vi "Word_Append_Or_Create_Table.vi"(7 "MS Office parameters":T1, 8 "error in (no error)":errorcluster, 9 "Data":string[][](array[string]), 10 "Column Headers":string[](array[string]), 11 "Report in":refnum<class "NI_report.lvclass">) -> (0 "error out":errorcluster, 3 "report out":refnum<class "NI_report.lvclass">)   [LabVIEW 2017, in "NI_ReportGenerationToolkit.lvlib"]
uses:
  <vilib>/addons/_office/NI_ReportGenerationToolkit.lvlib
  <vilib>/Utility/NIReport.llb/NI_report.lvclass
  <vilib>/Utility/NIReport.llb/Word/NI_Word.lvclass
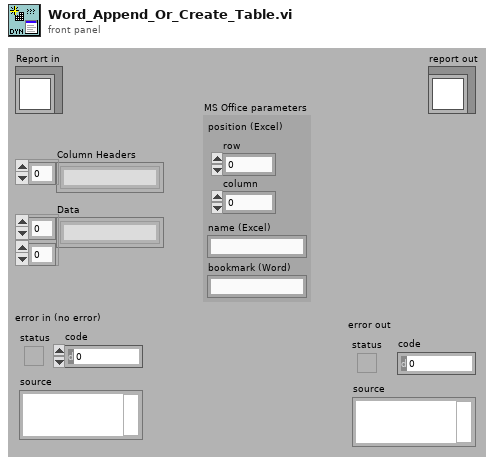
[diagram p1: front panel]
types:
  T1 = cluster{"position (Excel)":cluster{"row":i32, "column":i32}, "name (Excel)":string, "bookmark (Word)":string}
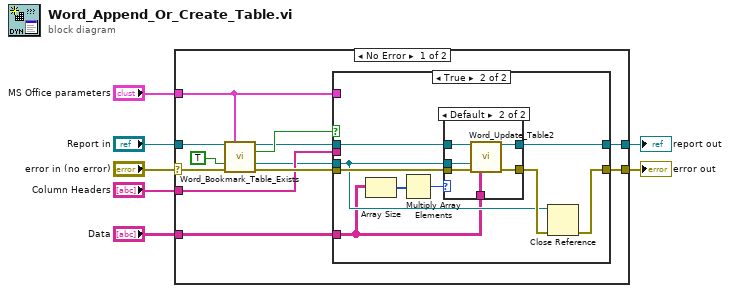
[diagram p0: block diagram]
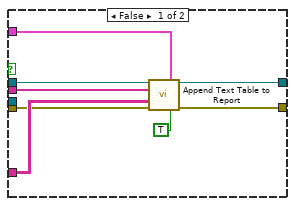
[diagram p2: hidden frame]
diagram:
  n1 = case shown="No Error" "error in (no error)" {
    selector: "error in (no error)" -> [w10 w45]
    tunnel: "MS Office parameters" -> [w16 _]
    tunnel: "Report in" -> [w15 w46]
    tunnel: "Column Headers" -> [w14 _]
    tunnel: "Data" -> [w13 _]
    tunnel: [w12 w45] -> w3
    tunnel: [w11 w46] -> w2
    frame No Error {
      n2 = call <vilib>:"Word_Bookmark_Table_Exists.vi"("report in"=w15, "MS Office parameters"=w16, "get table ref?"=TRUE ("Get Table Ref?"), "error in (no error)"=w10) -> ("report out"=w17:refnum<class "NI_report.lvclass">, "bookmark to existing table?"=w19:bool, "table ref"=w9:refnum<k7>, "error out"=w18:errorcluster)  [unwired: 8 in]
      n3 = case shown="True" w19 {
        tunnel: [w27 w34] -> w11
        tunnel: [w26 w32] -> w12
        tunnel: w13 -> [w24 w30]
        tunnel: w14 -> [w23 _]
        tunnel: w16 -> [w22 _]
        tunnel: w17 -> [w21 w35]
        tunnel: w18 -> [w20 w36]
        tunnel: w9 -> [_ w31]
        frame False {
          n4 = call-dynamic "Append Text Table to Report.vi"("report in"=w21, "MS Office parameters"=w22, "column headers"=w23, "text data"=w24, "error in (no error)"=w20, "show grid lines (YES)"=TRUE ("show grid lines")) -> ("report out"=w27:refnum<class "NI_report.lvclass">, "error out"=w26:errorcluster)  [unwired: 6 in, 2 out]
        }
        frame True {
          n5 = Array Size(array=w30) -> (size(s)=w28:i32[])
          n6 = Multiply Array Elements(1:w28) -> (0:w29:i32)
          n7 = case shown="Default" w29 {
            tunnel: w36 -> [w37 w44]
            tunnel: w35 -> [w38 w43]
            tunnel: [w38 w42] -> w34
            tunnel: w30 -> [_ w41]
            tunnel: [w37 w40] -> w33
            tunnel: w31 -> [_ w39]
            frame 0 {
            }
            frame Default {
              n8 = call <vilib>:"Word_Update_Table2.vi"("report in"=w43, "Table Ref"=w39, "error in (no error)"=w44, "value"=w41) -> ("report out"=w42:refnum<class "NI_report.lvclass">, "error out"=w40:errorcluster)  [unwired: 10 in]
            }
          }
          n9 = Close Reference(reference=w31, error in (no error)=w33) -> (error out=w32:errorcluster)
        }
      }
    }
    frame Error {
    }
  }
  "error out" <- w3
  "report out" <- w2
